vi "Check Signal with Limits.vi"(0 "Signal":T1, 5 "Positive Limit":T1, 7 "Negative Limit":T1, 11 "error in (no error)":errorcluster) -> (4 "In Range?":bool, 15 "error out":errorcluster)   [LabVIEW 2020]
doc: "VI checks for the Input Signal is \"In Range?\" within the positive and negative limit signals passed in the input."
uses:
  Plot Data.ctl
  <vilib>/gmath/NI_Gmath.lvlib
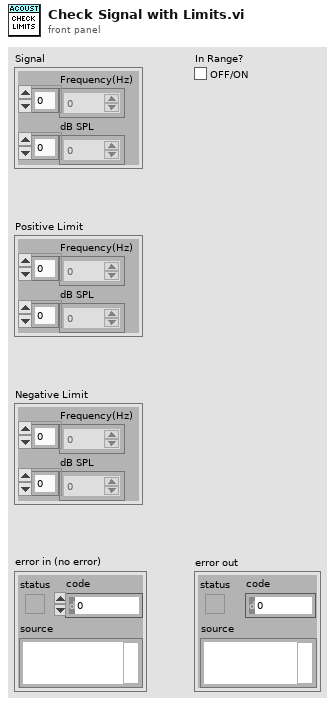
[diagram p1: front panel]
types:
  T1 = typedef "Plot Data.ctl" = cluster{"Frequency(Hz)":dbl[], "dB SPL":dbl[]}
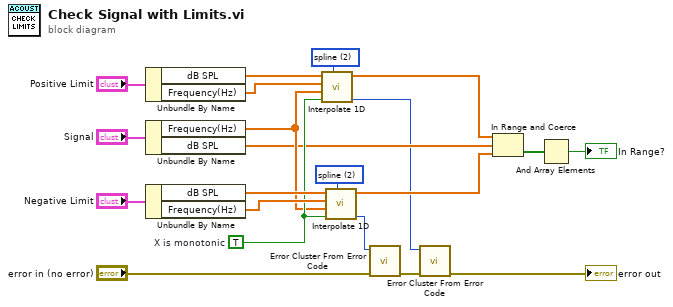
[diagram p0: block diagram]
diagram:
  w12 = TRUE  # X is monotonic
  w13 = 2 items=["nearest", "linear", "spline", "cubic Hermite", "Lagrange"] ("method")
  w18 = 2 items=["nearest", "linear", "spline", "cubic Hermite", "Lagrange"] ("method")
  n1 = Unbundle By Name("Positive Limit") -> ("dB SPL"=w17:dbl[], "Frequency(Hz)"=w16:dbl[])
  n2 = Unbundle By Name("Signal") -> ("Frequency(Hz)"=w11:dbl[], "dB SPL"=w9:dbl[])
  n3 = Unbundle By Name("Negative Limit") -> ("dB SPL"=w14:dbl[], "Frequency(Hz)"=w15:dbl[])
  n4 = call <vilib>:"Interpolate 1D.vi"("method"=w18, "X is monotonic"=w12, "xi"=w11, "X"=w16, "Y"=w17) -> ("error"=w1:i32, "yi"=w10:dbl[])  [unwired: 4 in, 1 out]
  n5 = call <vilib>:"Interpolate 1D.vi"("method"=w13, "X is monotonic"=w12, "xi"=w11, "X"=w15, "Y"=w14) -> ("error"=w4:i32, "yi"=w8:dbl[])  [unwired: 4 in, 1 out]
  n6 = call <vilib>:"Error Cluster From Error Code.vi"("error in (no error)"="error in (no error)", "error code (0)"=w4) -> ("error out"=w3:errorcluster)  [unwired: 7 in]
  n7 = call <vilib>:"Error Cluster From Error Code.vi"("error in (no error)"=w3, "error code (0)"=w1) -> ("error out"=→"error out":errorcluster)  [unwired: 7 in]
  n8 = In Range and Coerce(upper limit=w10, x=w9, lower limit=w8) -> (In Range?=w7:bool[])  [unwired: 1 out]
  n9 = And Array Elements(Boolean array=w7) -> (logical AND=→"In Range?":bool)
